vi "Test Tag Read Pictures Vorbis.vi"(8 "error in (no error)":errorcluster) -> (0 "error out":errorcluster, 3 "Pass?":bool)   [LabVIEW 2020]
uses:
  43f3824e-4ae3-4ff0-bba1-56c38b92c11b.vi
  G-Audio/Audio Files/Polymorphic VIs/Get Audio File Tags (Path).vi
  G-Audio/G-Audio.lvlib
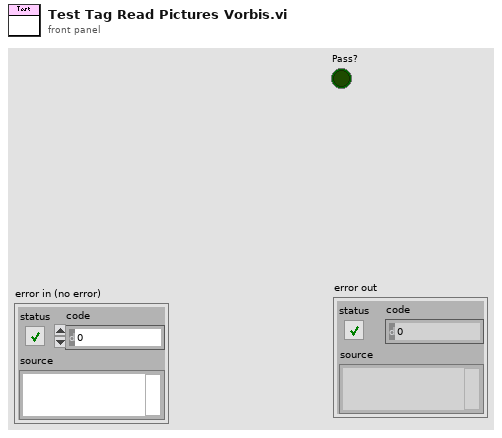
[diagram p1: front panel]
types:
  T1 = typedef "G-Audio.lvlib/Audio File Image.ctl" = cluster{"Type":T2, "Pixmap":T3}
  T2 = typedef "G-Audio.lvlib/Audio File Image Type.ctl" = enum32{"Other", "32x32 pixels 'file icon' (PNG only)", "Other file icon", "Cover (front)", "Cover (back)", "Leaflet page", "Media (e.g. label side of CD)", "Lead artist/lead performer/soloist", "Artist/performer", "Conductor", "Band/Orchestra", "Composer", "Lyricist/text writer", "Recording Location", "During recording", "During performance", "Movie/video screen capture", "A bright coloured fish", "Illustration", "Band/artist logotype", "Publisher/Studio logotype"}
  T3 = typedef "imagedata.ctl" = cluster{"image type":i32, "image depth":i32, "image":u8[], "mask":u8[], "colors":u32[], "Rectangle":cluster{"left":i16, "top":i16, "right":i16, "bottom":i16}}
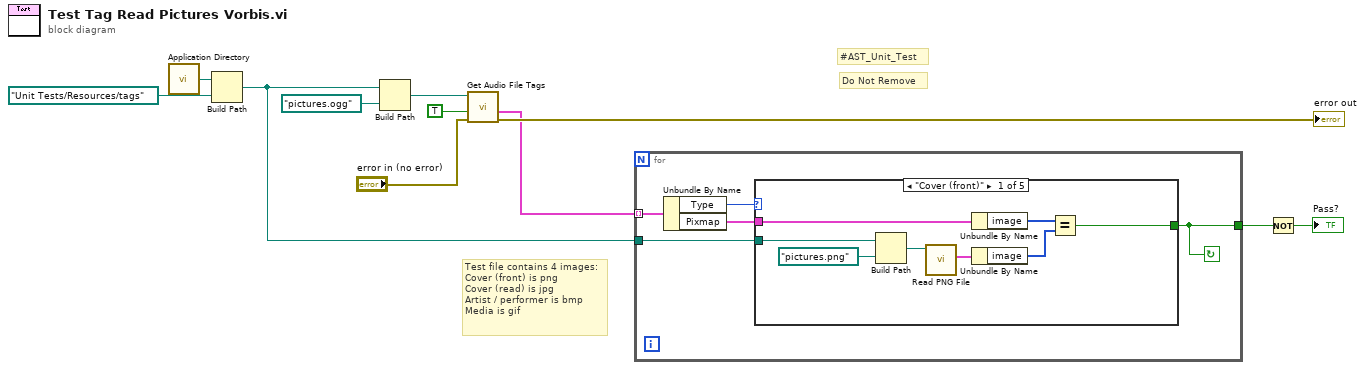
[diagram p0: block diagram]
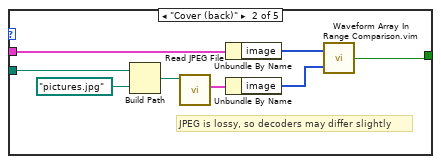
[diagram p2: hidden frame]
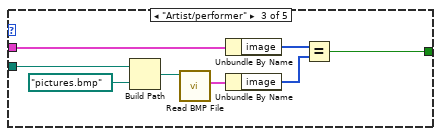
[diagram p3: hidden frame]
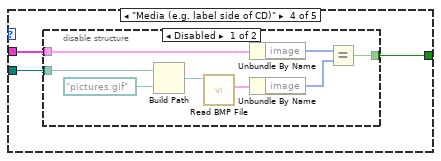
[diagram p4: hidden frame]
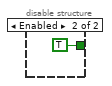
[diagram p5: hidden frame]
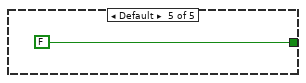
[diagram p6: hidden frame]
diagram:
  # "Test file contains 4 images:\nCover (front) is png\nCover (read) is jpg\nArtist / performer is bmp\nMedia is gif"
  # "Do Not Remove"
  # "#AST_Unit_Test"
  n1 = call <vilib>:"Application Directory.vi"() -> ("Application Directory"=w11:path)
  n2 = Build Path(base path=w11, name or relative path=path "Unit Tests/Resources/tags" ("Path")) -> (appended path=w3:path)
  n3 = Build Path(base path=w3, name or relative path=path "pictures.ogg") -> (appended path=w5:path)
  n4 = call-poly "Get Audio File Tags.vi"("error in (no error)"="error in (no error)", "Read Pictures? (F)"=TRUE, "Path In"=w5) -> ("error out"=→"error out":errorcluster, "Pictures"=w6:T1[])  [unwired: 5 in, 2 out]
  n5 = for {
    tunnel: w6 -> [w16] mode=indexing
    tunnel: w3 -> [w13]
    tunnel: [w12] -> w2
    stop <- w12 continue-if-true
    n6 = Unbundle By Name(w16) -> ("Type"=w15:T2, "Pixmap"=w14:T3)
    n7 = case shown="\"Cover (front)\"" w15 {
      tunnel: w14 -> [w24 w32 w40 w43 _]
      tunnel: w13 -> [w19 w30 w35 w41 _]
      tunnel: [w20 w25 w36 w42 FALSE] -> w12
      frame "Cover (front)" {
        n8 = Build Path(base path=w19, name or relative path=path "pictures.png") -> (appended path=w17:path)
        n9 = call <vilib>:"Read PNG File.vi"("path to PNG file"=w17) -> ("image data"=w23:T3)  [unwired: 8 in, 2 out]
        n10 = Unbundle By Name(w24) -> ("image"=w22:u8[])
        n11 = Unbundle By Name(w23) -> ("image"=w21:u8[])
        n12 = Equal?(x=w22, y=w21) -> (x = y?=w20:bool)
      }
      frame "Cover (back)" {
        # "JPEG is lossy, so decoders may differ slightly"
        n13 = Build Path(base path=w30, name or relative path=path "pictures.jpg") -> (appended path=w28:path)
        n14 = call <vilib>:"Read JPEG File.vi"("path to JPEG file"=w28) -> ("image data"=w31:T3)  [unwired: 8 in, 2 out]
        n15 = Unbundle By Name(w32) -> ("image"=w27:u8[])
        n16 = Unbundle By Name(w31) -> ("image"=w26:u8[])
        n17 = call "Waveform Array In Range Comparison.vim"("Expected Value"=w26, "Resulting Value"=w27) -> ("Comparison Result"=w25:bool)
      }
      frame "Artist/performer" {
        n18 = Build Path(base path=w35, name or relative path=path "pictures.bmp") -> (appended path=w33:path)
        n19 = call <vilib>:"Read BMP File.vi"("path to BMP file"=w33) -> ("image data"=w39:T3)  [unwired: 8 in, 2 out]
        n20 = Unbundle By Name(w40) -> ("image"=w38:u8[])
        n21 = Unbundle By Name(w39) -> ("image"=w37:u8[])
        n22 = Equal?(x=w38, y=w37) -> (x = y?=w36:bool)
      }
      frame "Media (e.g. label side of CD)" {
        n23 = disable-structure shown="Disabled" {
          disable-tunnel: w43 -> [w51 _]
          disable-tunnel: [w47 TRUE] -> w42
          disable-tunnel: w41 -> [w46 _]
          frame Disabled {
            n24 = Build Path(base path=w46, name or relative path=path "pictures.gif") -> (appended path=w44:path)
            n25 = call <vilib>:"Read BMP File.vi"("path to BMP file"=w44) -> ("image data"=w50:T3)  [unwired: 8 in, 2 out]
            n26 = Unbundle By Name(w51) -> ("image"=w49:u8[])
            n27 = Unbundle By Name(w50) -> ("image"=w48:u8[])
            n28 = Equal?(x=w49, y=w48) -> (x = y?=w47:bool)
          }
          frame Enabled {
          }
        }
      }
      frame Default {
      }
    }
  }
  n29 = Not(x=w2) -> (.not. x?=→"Pass?":bool)
